vi "IsPointSurrounded.vi"(10 "Position of Point":T1 {"North" format="%#_10f"; "East" format="%#_8f"}, 11 "Obstacle Array":refnum<class "Obstacle.lvclass">[](array[class])) -> (2 "IDs of Obstacles Surrounding Point":i32[](array[numeric]), 3 "Point is Surrounded":bool)   [LabVIEW 2013, in "Obstacle.lvclass"]
doc: "This checks through an array of obstacles and determines whether to point is surrounded by any obstacles. If it is, it lists the IDs of all obstacles surrounding the point.\n\nEric Schneider, August 2014"
uses:
  Obstacle.lvclass
  Data/TypeDefs/UTM Location.ctl
panel:
  in  "Number of angles to check":i32=360
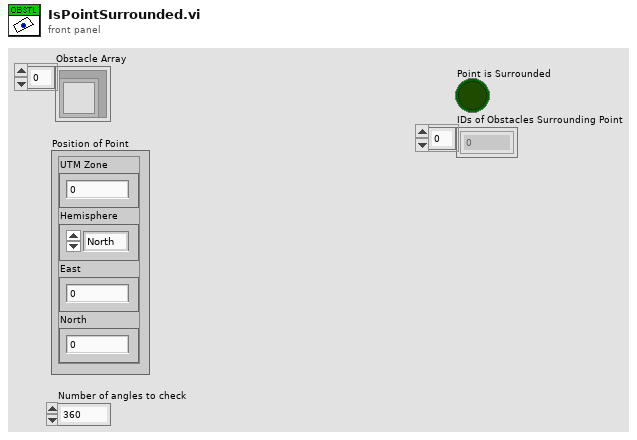
[diagram p1: front panel]
types:
  T1 = typedef "UTM Location.ctl" = cluster{"UTM Zone":dbl, "Hemisphere":enum16{"North", "South"}, "East":dbl, "North":dbl}
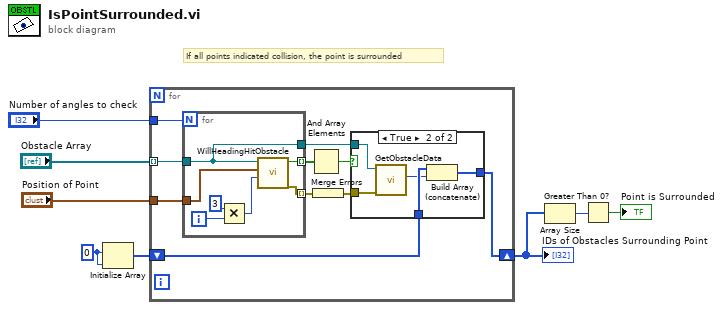
[diagram p0: block diagram]
diagram:
  w5 = 0
  # "If all points indicated collision, the point is surrounded"
  n1 = Initialize Array(w5, w5) -> (w4:i32[])
  n2 = for {
    tunnel: "Obstacle Array" -> [w17] mode=indexing
    tunnel: "Position of Point" -> [w16]
    tunnel: "Number of angles to check" -> [w18]
    shift-right: [w9] -> w3
    shift-left: w4 -> [w10]
    n3 = for {
      N: w18 -> [_]
      tunnel: w17 -> [w29]
      tunnel: w16 -> [w31]
      tunnel: [w30] -> w15 mode=indexing
      tunnel: [w29] -> w13
      tunnel: [w28] -> w12 mode=indexing
      i -> [w27]
      n4 = Multiply(x=3, y=w27) -> (x*y=w25:i32)
      n5 = call "WillHeadingHitObstacle.vi"("Heading"=w25, "Boat"=w31, "Obstacle.lvclass"=w29) -> ("error out"=w28:errorcluster, "Any intersecting obstacles?"=w30:bool)  [unwired: 7 in]
    }
    n6 = And Array Elements(Boolean array=w15) -> (logical AND=w14:bool)
    n7 = Merge Errors(w12) -> (w11:errorcluster)
    n8 = case shown="True" w14 {
      tunnel: w13 -> [_ w24]
      tunnel: w11 -> [_ w23]
      tunnel: [w19 w20] -> w9
      tunnel: w10 -> [w19 w22]
      frame False {
      }
      frame True {
        n9 = call "GetObstacleData.vi"("error in (no error)"=w23, "Obstacle.lvclass"=w24) -> ("ID#"=w21:i32)  [unwired: 6 in, 3 out]
        n10 = Build Array (concatenate)(w22, w21) -> (w20:i32[])
      }
    }
  }
  "IDs of Obstacles Surrounding Point" <- w3
  n11 = Array Size(array=w3) -> (size(s)=w2:i32)
  n12 = Greater Than 0?(x=w2) -> (x > 0?=→"Point is Surrounded":bool)
